vi "REC STOP.vi"(0 "System no.":i32=1 min=1 max=4 step=1, 2 "RecorderIDs":string[](array[string]), 5 "error in":errorcluster) -> (19 "error out":errorcluster)   [LabVIEW 2020]
doc: "REC STOP (Stop Data Recorder)\n\nDescription\nStops a data recorder.\nIt is necessary to stop a data recorder before you can change its configuration (recording rate, \ntrigger, variable to be recorded). Stopping the data recorder will end the current recording and \ndeactivate the set trigger.\nStopping the data recorder switches its state from \"WAIT\" or \"RUN\" to \"CFG\". For more details, \nsee the state diagram for the data recorder (p. 110). The state of the data recorder can be \nqueried with REC? STATE (p. 47). \n\nFormat\nREC STOP <RecorderID>\n\nArguments\n<RecorderID>\nData recorder to be stopped; to be specified as alias (p. 94) \nThe available data recorders can be queried with USG? SYS (p. 80). \nPossible values: REC_1 to RECn, where n = number of data recorders in the controller\n\nResponse\nnone\n\nExample\n>> REC STOP REC_1\n>> REC STOP REC_2\n\nNotes\nFor further details, see \"Data Recorder - GCS 3.0\" (p. 107). \n\nUser command level\nUSR"
panel:
  # "REC STOP (Stop Data Recorder)\n\nStops a data recorder.\nIt is necessary to stop a data recorder before you can change its configuration (recording rate, trigger, variable to be recorded). Stopping the data recorder will end the current recording and \ndeactivate the set trigger.\nStopping the data recorder switches its state from \"WAIT\" or \"RUN\" to \"CFG\". For more details,  see the state diagram for the data recorder. The state of the data recorder can be queried with REC? STATE."
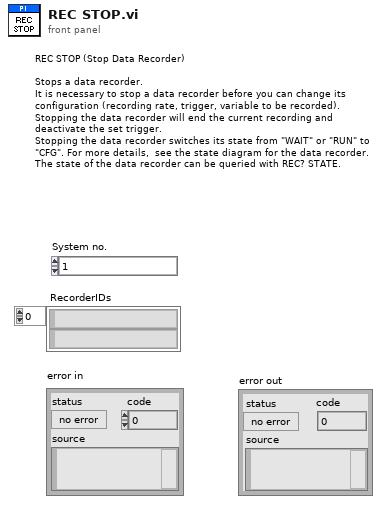
[diagram p1: front panel]
types:
  T1 = typedef "Syntax.ctl" = enum16{"GCS 1.0", "GCS 2.0", "GCS 3.0"}
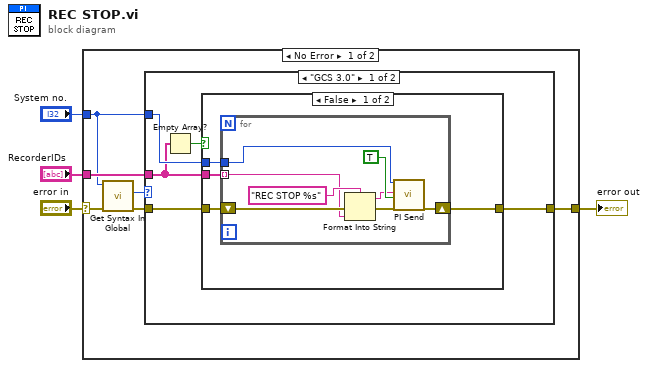
[diagram p0: block diagram]
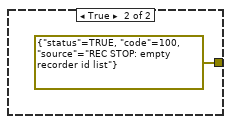
[diagram p2: hidden frame]
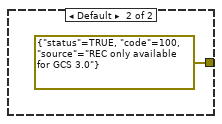
[diagram p3: hidden frame]
diagram:
  n1 = case shown="No Error" "error in" {
    selector: "error in" -> [w10 w30]
    tunnel: [w7 w30] -> w1
    tunnel: "RecorderIDs" -> [w6 _]
    tunnel: "System no." -> [w5 _]
    frame No Error {
      n2 = call "Get Syntax In Global.vi"("error in"=w10, "System no."=w5) -> ("error out"=w8:errorcluster, "Syntax"=w9:T1)  [unwired: 8 in]
      n3 = case shown="\"GCS 3.0\"" w9 {
        tunnel: w8 -> [w13 _]
        tunnel: [w14 errorcluster {"status"=TRUE, "code"=100, "source"="REC only available for GCS 3.0"} ("error out")] -> w7
        tunnel: w6 -> [w12 _]
        tunnel: w5 -> [w15 _]
        frame "GCS 3.0" {
          n4 = Empty Array?(array=w12) -> (empty?=w11:bool)
          n5 = case shown="False" w11 {
            tunnel: w15 -> [w19 _]
            tunnel: w12 -> [w18 _]
            tunnel: [w17 errorcluster {"status"=TRUE, "code"=100, "source"="REC STOP: empty recorder id list"} ("error out")] -> w14
            tunnel: w13 -> [w16 _]
            frame False {
              n6 = for {
                shift-right: [w27] -> w17
                shift-left: w16 -> [w21]
                tunnel: w19 -> [w26]
                tunnel: w18 -> [w20] mode=indexing
                n7 = Format Into String(format string="REC STOP %s", error in=w21, w20) -> (resulting string=w23:string, error out=w24:errorcluster)  [unwired: 1 in]
                n8 = call "PI Send.vi"("System no."=w26, "String to send"=w23, "Attach termination char.?"=TRUE, "error in"=w24) -> ("error out"=w27:errorcluster)  [unwired: 2 in, 13 out]
              }
            }
            frame True {
            }
          }
        }
        frame Default {
        }
      }
    }
    frame Error {
    }
  }
  "error out" <- w1
